vi "Run.vi"(7 "Team Index":i32, 8 "Column":i32, 9 "Row":i32, 10 "View":i32[](array[numeric]) caption="View (Team Index, -1: empty)", 11 "Great Wall In":refnum<class "Great Wall.lvclass">) -> (0 "Replicated":refnum<class "Square.lvclass">, 1 "Direction":T1, 2 "Action":T2, 3 "Square Out":refnum<class "Square.lvclass">)   [LabVIEW 2020, in "Great Wall.lvclass"]
uses:
  Great Wall.lvclass
  C:/dev/IlluminatedG/sol-squarebattle/Square/Square.lvclass
  Square/Square.lvclass
  Type Defs/Action Enum.ctl
  Type Defs/Direction Enum.ctl
  Great Wall.lvclass/Great Wall.ctl
  Wall State.ctl
  Wall State Enum.ctl
  Private Data.ctl
  Type Defs/SB Type Defs.lvlib
  DS Square Library/DS Square.lvlib
panel:
  # "NW\nN\nNE\nE\nSE\nS\nSW\nW"
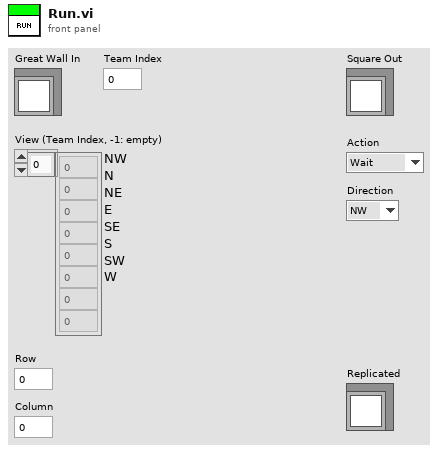
[diagram p1: front panel]
types:
  T1 = typedef "SB Type Defs.lvlib/Direction Enum.ctl" = enum16{"NW", "N", "NE", "E", "SE", "S", "SW", "W"}
  T2 = typedef "SB Type Defs.lvlib/Action Enum.ctl" = enum16{"Wait", "Move", "Attack", "Replicate"}
  T3 = typedef "Great Wall.lvclass/Private Data.ctl" = cluster{"wall 1":T4, "wall 2":T4, "start row":i32, "start col":i32, "state update round":i32}
  T4 = typedef "Great Wall.lvclass/Wall State.ctl" = cluster{"state":T5, "direction":T1, "index":i32}
  T5 = typedef "Great Wall.lvclass/Wall State Enum.ctl" = enum16{"Under Construction", "Hold", "Advance 1", "Advance 2", "Retreat"}
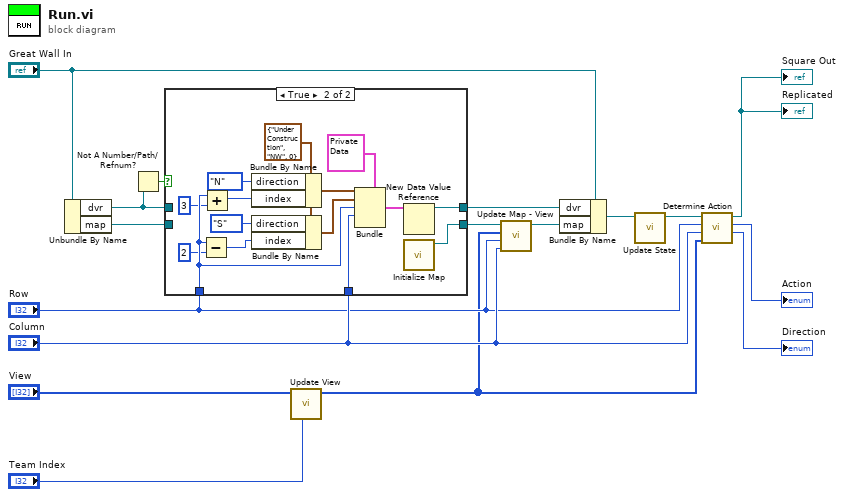
[diagram p0: block diagram]
diagram:
  n1 = Unbundle By Name("Great Wall In") -> ("dvr"=w16:refnum<data-value>, "map"=w14:refnum<data-value>)
  n2 = Not A Number/Path/Refnum?(number/path/refnum=w16) -> (NaN/Path/Refnum?=w17:bool)
  n3 = case shown="True" w17 {
    tunnel: "Row" -> [_ w22]
    tunnel: [w19 w27] -> w12
    tunnel: w16 -> [w19 _]
    tunnel: "Column" -> [_ w25]
    tunnel: w14 -> [w18 _]
    tunnel: [w18 w24] -> w13
    frame False {
    }
    frame True {
      w33 = T4 {"state"=enum."Under Construction", "direction"=enum."NW", "index"=0} ("wall")
      n4 = Subtract(x=w22, y=2) -> (x-y=w31:i32)
      n5 = Add(x=w22, y=3) -> (x+y=w23:i32)
      n6 = Bundle By Name(cluster=w33, "direction"=Direction_Enum."N", "index"=w23) -> (w30:T4)
      n7 = Bundle By Name(cluster=w33, "direction"=Direction_Enum."S", "index"=w31) -> (w29:T4)
      n8 = Bundle(cluster=T3 {"wall 1"={"state"=enum."Under Construction", "direction"=enum."NW", "index"=0}, "wall 2"={"state"=enum."Under Construction", "direction"=enum."NW", "index"=0}, "start row"=0, "start col"=0, "state update round"=0} ("private data"), "wall 1"=w30, "wall 2"=w29, "start row"=w22, "start col"=w25) -> (w28:T3)  [unwired: 1 in]
      n9 = New Data Value Reference(data value=w28) -> (data value reference=w27:refnum<data-value>)  [unwired: 1 in, 1 out]
      n10 = call "Initialize Map.vi"() -> ("map"=w24:refnum<data-value>)  [unwired: 11 in]
    }
  }
  n11 = call "Update View.vi"("Team Index"="Team Index", "View"="View") -> ("View out"=w1:i32[])  [unwired: 9 in]
  n12 = call "Update Map - View.vi"("Column"="Column", "Row"="Row", "Updated View"=w1, "map in"=w13) -> ("map out"=w11:refnum<data-value>)  [unwired: 7 in]
  n13 = Bundle By Name(cluster="Great Wall In", "dvr"=w12, "map"=w11) -> (w10:refnum<class "Great Wall.lvclass">)
  n14 = call "Update State.vi"("Great Wall in"=w10) -> ("Great Wall out"=w9:refnum<class "Great Wall.lvclass">)  [unwired: 10 in]
  n15 = call "Determine Action.vi"("Updated View"=w1, "Column"="Column", "Row"="Row", "Great Wall in"=w9) -> ("Direction"=→"Direction":T1, "Action"=→"Action":T2, "Great Wall out"=→"Square Out" →"Replicated":refnum<class "Great Wall.lvclass">)  [unwired: 5 in]
